vi "Acquisition-Error handler.vi"(8 "error in (no error)":errorcluster, 11 "Message Queues":T1) -> (0 "error out":errorcluster)   [LabVIEW 2020]
uses:
  User Interface/Queue/Message Queue/Typedefs/All Message Queues.ctl
  User Interface/Queue/Message Queue/Typedefs/Message Cluster.ctl
  Typedefs/Logging queue element.ctl
  Typedefs/Imaging Protocols enum.ctl
  Typedefs/Frame Size.ctl
  Typedefs/Acquired points count.ctl
  <vilib>/Utility/error.llb/DialogType.ctl
  Typedefs/Top level VI states.ctl
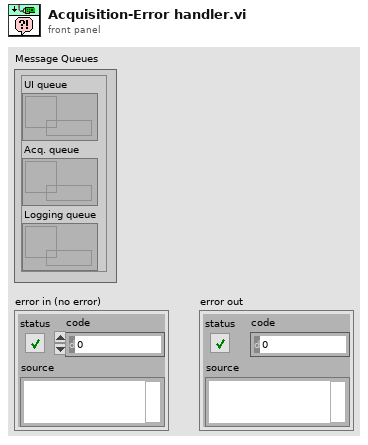
[diagram p1: front panel]
types:
  T1 = typedef "All Message Queues.ctl" = cluster{"UI queue":refnum<queue>, "Acq. queue":refnum<queue>, "Logging queue":refnum<queue>}
  T2 = typedef "Top level VI states.ctl" = enum16{"None", "Initialise UI", "<STACK PROTOCOL STATES>", "AOL Zstack-START", "AOL Zstack-STOP", "Motor Zstack-START", "Motor Zstack-STOP", "<ACQUISITION PROTOCOL STATES> ", "Functional Acquisition-START", "Functional Acquisition-STOP", "Single Plane Acquisition-START", "Single Plane Acquisition-STOP", "Volume Acquisition-START", "Volume Acquisition-STOP", "<LIVE IMAGING PROTOCOL STATES>", "Live Imaging-START", "Live Imaging-STOP", "Live Plane Imaging-START", "Live Plane Imaging-STOP", "Live Volume Imaging-START", "Live Volume Imaging-STOP", "<MOVEMENT CORRECTION PROTOCOL STATES>", "EXIT"}
  T3 = typedef "AOL_Globals.ctl" = cluster{"Imaging Protocol":T4, "Number of POI":u16, "Number of Miniscans":u16, "Number of Trials":u16, "Number of Cycles ":u64, "# Averaged Frames":u16, "Laser power (%)":u8, "Pockels (V)":dbl, "Acquisition Length (sec)":dbl, "Fill time (us)":dbl, "POI Dwell time (us)":dbl, "Miniscan Dwell time per pixel (us)":dbl, "PMT 1":dbl, "PMT 2":dbl, "Back Apperture (mA)":dbl, "Frame Size":T5, "Center Frequency":dbl, "Field of View (norm)":dbl, "DwellTime (us)":dbl, "Wavelength (nm)":dbl, "Zoom":dbl, "AOL Z":dbl, "AOL Mode":T6, "GridXY":dbl, "GridZ":dbl, "TriggerPeriod (sec)":dbl, "Number of Pixels in Miniscan":u16, "Experiment folder path":path, "X centre":dbl, "Y centre":dbl, "Angle (degrees)":dbl, "Plane Mode":T7, "Threshold":u16[], "Regenerate Chirps":bool, "Rectangle ROI length (pixels)":u16, "Rectangle ROI height (pixels)":u16, "AOD fill":u16, "StartupDelay":i32, "Samples Wait after Trigger":u16, "Slip Cycle":u32, "Add Cycle":bool, "Functional Mode":T8, "Z Start":dbl, "Z Stop":dbl, "# Planes":i32, "Total Pixels":i32, "Variable Miniscan Pixels":u16[], "Use Variable Length":bool, "Use Variable Resolution":bool, "Laser power (%) at Z Start":u8, "Laser power (%) at Z Stop":u8, "Ref Z Step":i8, "Ref Dwell Time (us)":dbl, "Field of View (um)":dbl}
  T4 = typedef "Imaging Protocols enum.ctl" = enum16{"AOL Z-Stack", "Motor Z Stack", "Functional Acquisition", "Single Plane Acquisition", "Volume Acquisition", "Live Imaging", "Live Plane Imaging", "Live Volume Imaging"}
  T5 = typedef "Frame Size.ctl" = u16
  T6 = typedef "AOL modes.ctl" = enum16{"Raster", "Structural", "Pointing", "Mini Scan", "Alignment"}
  T7 = typedef "Plane Mode.ctl" = u16
  T8 = typedef "Functional Mode.ctl" = enum16{"Point", "Line", "Patch", "Plane", "Volume"}
  T9 = typedef "DialogType.ctl" = u16
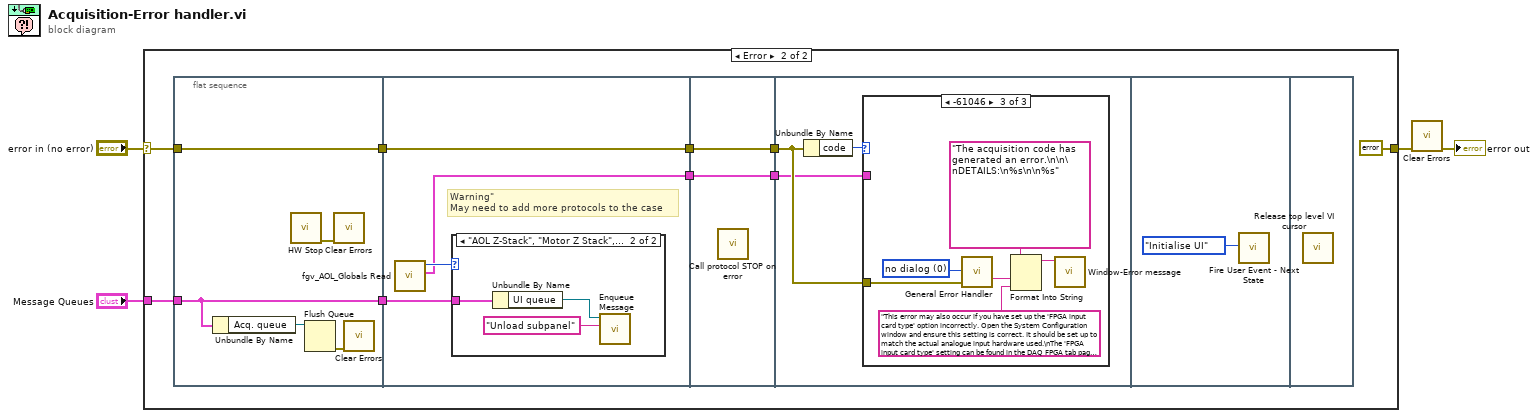
[diagram p0: block diagram]
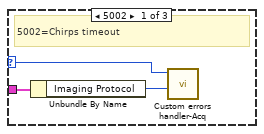
[diagram p4: hidden frame]
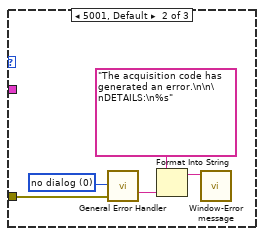
[diagram p5: hidden frame]
diagram:
  n1 = case shown="Error" "error in (no error)" {
    selector: "error in (no error)" -> [_ w9]
    tunnel: [_ errorcluster {"status"=FALSE, "code"=0, "source"=""} ("error out")] -> w3
    tunnel: "Message Queues" -> [_ w11]
    frame No Error {
    }
    frame Error {
      n2 = flat-sequence {
        tunnel: [w16] -> w12
        tunnel: w11 -> [w16]
        tunnel: [w18] -> w10
        tunnel: w9 -> [w18]
        tunnel: w12 -> [w22]
        tunnel: [w21] -> w8
        tunnel: w10 -> [w21]
        tunnel: [w19] -> w5
        tunnel: w8 -> [w27]
        tunnel: [w27] -> w7
        tunnel: [w26] -> w6
        tunnel: w5 -> [w26]
        tunnel: w7 -> [w29]
        tunnel: w6 -> [w28]
        frame #0 {
          n3 = Unbundle By Name(w16) -> ("Acq. queue"=w15:refnum<queue>)
          n4 = call "HW Stop.vi"() -> ("error out"=w17:errorcluster)  [unwired: 11 in]
          n5 = Flush Queue(queue=w15) -> (error out=w14:errorcluster)  [unwired: 1 in, 2 out]
          n6 = call <vilib>:"Clear Errors.vi"("error in (no error)"=w17) -> ()  [unwired: 5 in, 2 out]
          n7 = call <vilib>:"Clear Errors.vi"("error in (no error)"=w14) -> ()  [unwired: 5 in, 2 out]
        }
        frame #1 {
          # "Warning\"\nMay need to add more protocols to the case"
          n8 = call "fgv_AOL_Globals Read.vi"() -> ("AOL_Globals"=w19:T3, "Imaging Protocol"=w20:T4)  [unwired: 9 in, 1 out]
          n9 = case shown="\"AOL Z-Stack\", \"Motor Z Stack\", \"Single Plane Acquisition\"" w20 {
            tunnel: w22 -> [_ w25]
            frame Default {
            }
            frame "AOL Z-Stack", "Motor Z Stack", "Single Plane Acquisition" {
              n10 = Unbundle By Name(w25) -> ("UI queue"=w23:refnum<queue>)
              n11 = call "Enqueue Message.vi"("Message"="Unload subpanel", "Queue"=w23) -> ()  [unwired: 8 in, 2 out]
            }
          }
        }
        frame #2 {
          n12 = call "Call protocol STOP on error.vi"() -> ()  [unwired: 11 in, 1 out]
        }
        frame #3 {
          n13 = Unbundle By Name(w29) -> ("code"=w30:i32)
          n14 = case shown="-61046" w30 {
            selector: w30 -> [w33 _ _]
            tunnel: w29 -> [_ w37 w43]
            tunnel: w28 -> [w32 _ _]
            frame 5002 {
              # "5002=Chirps timeout"
              n15 = Unbundle By Name(w32) -> ("Imaging Protocol"=w31:T4)
              n16 = call "Custom errors handler-Acq.vi"("Imaging Protocol"=w31, "code"=w33) -> ()  [unwired: 10 in]
            }
            frame 5001, Default {
              w38 = T9 0 items=["no dialog", "OK message", "continue or stop message", "OK message + warnings", "continue/stop + warnings"] ("type of dialog (OK msg:1)")
              n17 = call <vilib>:"General Error Handler.vi"("type of dialog (OK msg:1)"=w38, "error in (no error)"=w37) -> ("message"=w34:string)  [unwired: 9 in, 4 out]
              n18 = Format Into String(format string="The acquisition code has generated an error.\n\n\nDETAILS:\n%s" ("Error Source"), w34) -> (resulting string=w36:string)  [unwired: 2 in, 1 out]
              n19 = call "Window-Error message.vi"("Message"=w36) -> ()  [unwired: 10 in, 1 out]
            }
            frame -61046 {
              w44 = T9 0 items=["no dialog", "OK message", "continue or stop message", "OK message + warnings", "continue/stop + warnings"] ("type of dialog (OK msg:1)")
              n20 = call <vilib>:"General Error Handler.vi"("type of dialog (OK msg:1)"=w44, "error in (no error)"=w43) -> ("message"=w40:string)  [unwired: 9 in, 4 out]
              n21 = Format Into String(format string="The acquisition code has generated an error.\n\n\nDETAILS:\n%s\n\n%s" ("Error Source"), w40, "This error may also occur if you have set up the 'FPGA input card type' option incorrectly. Open the System Configuration window and ensure this setting is correct. It should be set up to match the actual analogue input hardware used.\nThe 'FPGA input card type' setting can be found in the DAQ FPGA tab page in the System Configuration window.\n" ("Error Source")) -> (resulting string=w42:string)  [unwired: 2 in, 1 out]
              n22 = call "Window-Error message.vi"("Message"=w42) -> ()  [unwired: 10 in, 1 out]
            }
          }
        }
        frame #4 {
          n23 = call "Fire User Event - Next State.vi"("\"UI Handler loop\" case to execute"=Top_level_VI_states."Initialise UI" ("State")) -> ()  [unwired: 10 in, 1 out]
        }
        frame #5 {
          n24 = call "Release top level VI cursor.vi"() -> ()  [unwired: 12 in]
        }
      }
    }
  }
  n25 = call <vilib>:"Clear Errors.vi"("error in (no error)"=w3) -> ("error out"=→"error out":errorcluster)  [unwired: 5 in, 1 out]
